vi "throttle from query.vi"() -> ()   [LabVIEW 2012]
panel:
  out "Throttle Q":bool
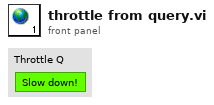
[diagram p1: front panel]
diagram:
